vi "PCO_Save.vi"(6 "Save as...":enum16{".tiff", ".mat", "Both"}(ring), 7 "PCO_Config":T1={"Exposure time (s)"=0.01, "TriggerMode"=0, "ROI X0"=1, "ROI Y0"=1, "ROI X1"=2048, "ROI Y1"=2048, "Binning"=1} {"TriggerMode" items=["auto sequence", "software trigger", "external exposure start", "external exposure control"]}, 8 "entrée d'erreur (pas d'erreur)":errorcluster, 9 "raw_image_list (U16)":u16[][][](array[numeric]), 11 "SavePath":path=path "C:/Users/Sebastien/Documents/GitHub/LABVIEW_SEMO_TOMO/Data") -> (0 "sortie d'erreur":errorcluster={"status"=TRUE, "code"=1430, "source"="Créer un dossier dans PCO_Save.vi<APPEND>\numents\\GitHub\\LABVIEW_SEMO_TOMO\\Data\\20260708"})   [LabVIEW 2026]
uses:
  Controls/PCO_Config.ctl
panel:
  out "chaîne concaténée":string="python C:\\Users\\Sebastien\\Documents\\GitHub\\LABVIEW_SEMO_TOMO\\Labview_code\\v0.5\\SubVIs\\PCO\\PCO_assemble_tiff_stack.py \"C:\\Users\\Sebastien\\Documents\\GitHub\\LABVIEW_SEMO_TOMO\\Labview_code\\v0.5\\SubVIs\\PCO\\Filenames.csv\" --format tiff --delete-originals"
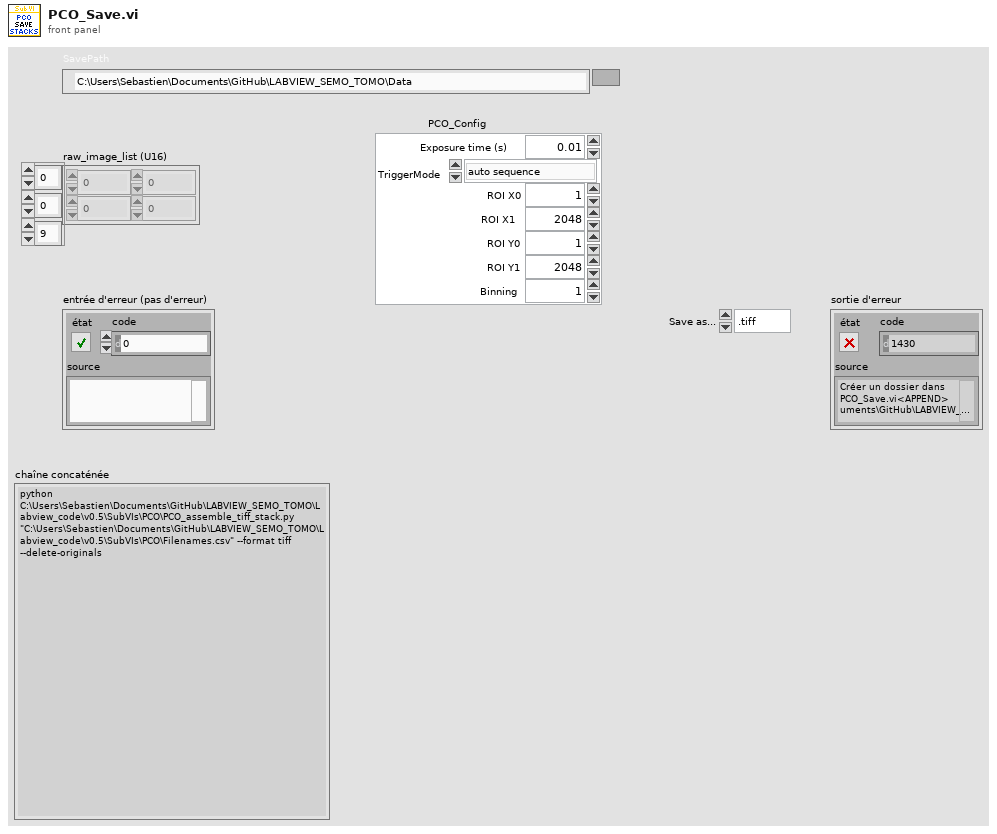
[diagram p1: front panel]
types:
  T1 = typedef "PCO_Config.ctl" = cluster{"Exposure time (s)":dbl, "TriggerMode":u16, "ROI X0":u16, "ROI Y0":u16, "ROI X1":u16, "ROI Y1":u16, "Binning":u8}
  T2 = enum16{"big-endian, network order", "native, host order", "little-endian"}
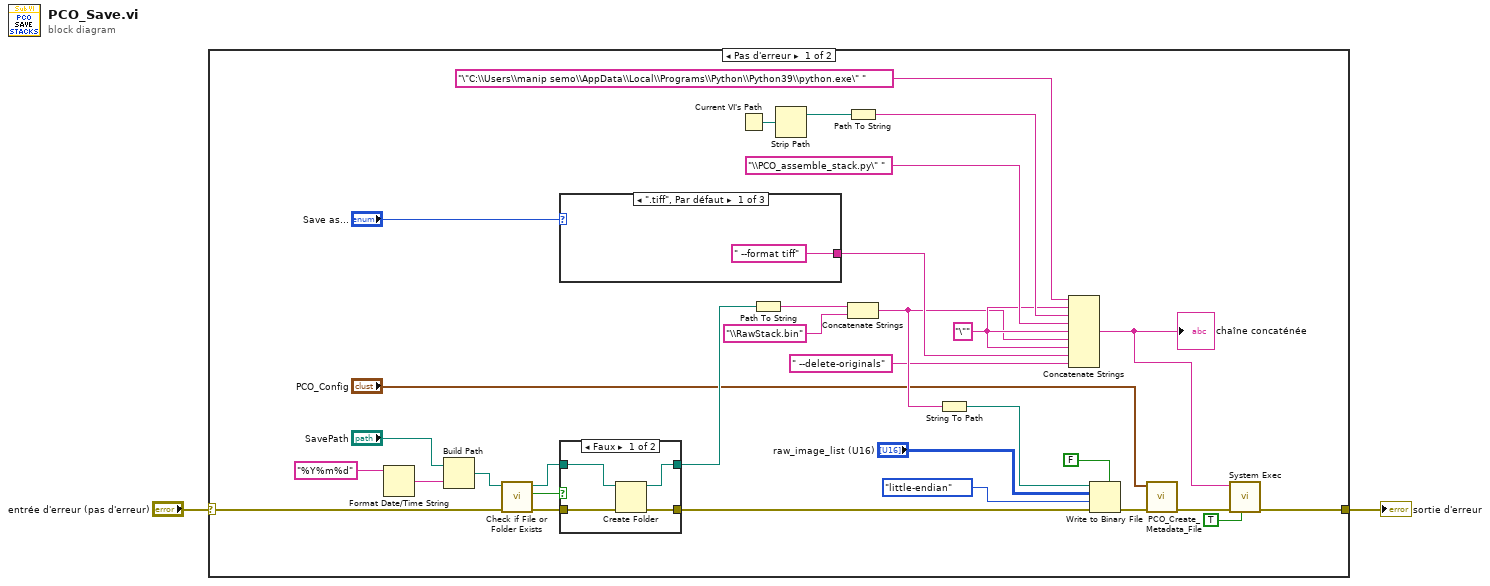
[diagram p0: block diagram]
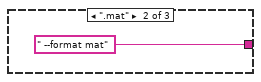
[diagram p2: hidden frame]
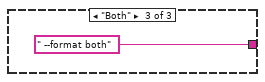
[diagram p3: hidden frame]
diagram:
  n1 = case shown="Pas d'erreur" "entrée d'erreur (pas d'erreur)" {
    selector: "entrée d'erreur (pas d'erreur)" -> [w22 w44]
    tunnel: [w27 w44] -> w2
    frame No Error {
      w15 = "\"" ("chaîne")
      n2 = Format Date/Time String(time format string (%c)="%Y%m%d" ("chaîne de format de l'heure (%c)")) -> (date/time string=w23:string)  [unwired: 2 in]
      n3 = Build Path(base path="SavePath", name or relative path=w23) -> (appended path=w21:path)
      n4 = call <vilib>:"Check if File or Folder Exists.vi"("error in (no error)"=w22, "path"=w21) -> ("error out"=w20:errorcluster, "file or folder exists?"=w18:bool, "dup path"=w19:path)  [unwired: 7 in]
      n5 = case shown="\".tiff\", Par défaut" "Save as..." {
        tunnel: [" --format tiff" ("chaîne") " --format mat" ("chaîne") " --format both" ("chaîne")] -> w16
        frame ".tiff", Default {
        }
        frame ".mat" {
        }
        frame "Both" {
        }
      }
      n6 = case shown="Faux" w18 {
        tunnel: [w41 w42] -> w9
        tunnel: [w38 w43] -> w13
        tunnel: w20 -> [w40 w43]
        tunnel: w19 -> [w39 w42]
        frame False {
          n7 = Create Folder(path (use dialog)=w39, error in=w40) -> (created path=w41:path, error out=w38:errorcluster)  [unwired: 1 in, 1 out]
        }
        frame True {
        }
      }
      n8 = Current VI's Path() -> (path=w30:path)
      n9 = Path To String(path=w9) -> (string=w8:string)
      n10 = Strip Path(path=w30) -> (stripped path=w29:path)  [unwired: 1 out]
      n11 = Path To String(path=w29) -> (string=w33:string)
      n12 = Concatenate Strings(w8, "\\RawStack.bin" ("chaîne")) -> (w6:string)
      n13 = String To Path(string=w6) -> (path=w7:path)
      n14 = Concatenate Strings("\"C:\\Users\\manip semo\\AppData\\Local\\Programs\\Python\\Python39\\python.exe\" " ("chaîne"), w15, w33, "\\PCO_assemble_stack.py\" " ("chaîne"), w15, w6, w15, w16, " --delete-originals" ("chaîne")) -> (w31:string)
      "chaîne concaténée" <- w31
      n15 = Write to Binary File(file (use dialog)=w7, data="raw_image_list (U16)", error in=w13, 5:FALSE ("ajouter une taille de tableau ou de chaîne ? (V)"), 9:T2."little-endian" ("ordre des octets (0 : big-Endian, network order)")) -> (error out=w14:errorcluster)  [unwired: 1 in, 2 out]
      n16 = call "PCO_Create_Metadata_File.vi"("entrée d'erreur"=w14, "PCO_Config"="PCO_Config") -> ("sortie d'erreur"=w26:errorcluster)  [unwired: 9 in]
      n17 = call <vilib>:"System Exec.vi"("run minimized? (F)"=TRUE, "error in (no error)"=w26, "command line"=w31) -> ("error out"=w27:errorcluster)  [unwired: 5 in, 3 out]
    }
    frame Error {
    }
  }
  "sortie d'erreur" <- w2
